vi "STM Read Meta Data (UDP Clst).vi"(6 "Options":T4={"Ignore Timeout Error"=TRUE, "timeout ms (1000)"=1000, "max size (548)"=548}, 8 "error in":errorcluster, 11 "Connection Info In":T2) -> (0 "error out":errorcluster, 1 "Meta data":T1[](array[typedef]), 3 "Connection Info Out":T2, 4 "data info":T3)   [LabVIEW 2014, in "QwaveSys Raspberry Pi Library.lvlib"]
doc: "This VI reads the meta data information from a remote computer. Use this VI to retrieve the variable names and types that a remote computer exports.\n\nThis VI parses the data and returns a cluster containing the meta data information."
uses:
  QwaveSys Raspberry Pi Library.lvlib
  stm_UDP Read Options.ctl
  stm_UDP Data Info.ctl
  stm_UDP Connection Info.ctl
  _SubVIs/stm_MetaDataElement.ctl
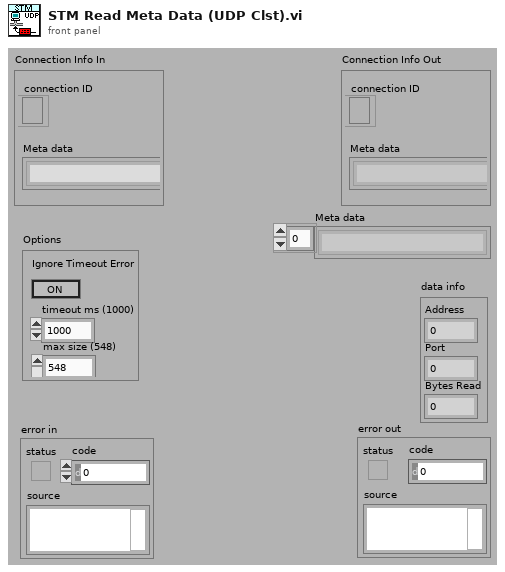
[diagram p1: front panel]
types:
  T1 = typedef "QwaveSys Raspberry Pi Library.lvlib/stm_MetaDataElement.ctl" = string
  T2 = typedef "QwaveSys Raspberry Pi Library.lvlib/stm_UDP Connection Info.ctl" = cluster{"connection ID":refnum<k16>, "Meta data":T1[]}
  T3 = typedef "QwaveSys Raspberry Pi Library.lvlib/stm_UDP Data Info.ctl" = cluster{"Address":u32, "Port":u16, "Bytes Read":i32}
  T4 = typedef "QwaveSys Raspberry Pi Library.lvlib/stm_UDP Read Options.ctl" = cluster{"Ignore Timeout Error":bool, "timeout ms (1000)":i32, "max size (548)":i32}
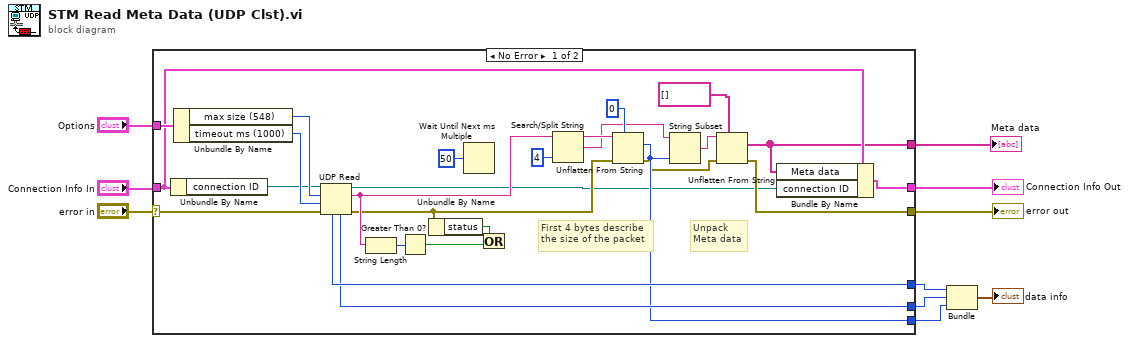
[diagram p0: block diagram]
diagram:
  n1 = case shown="No Error" "error in" {
    selector: "error in" -> [w35 w37]
    tunnel: [w12 _] -> w1
    tunnel: [w36 w37] -> w10
    tunnel: "Connection Info In" -> [w15 w38]
    tunnel: [w16 w38] -> w2
    tunnel: [w28 _] -> w8
    tunnel: [w27 _] -> w7
    tunnel: [w21 _] -> w6
    tunnel: "Options" -> [w17 _]
    frame No Error {
      # "First 4 bytes describe\nthe size of the packet"
      # "Unpack\nMeta data"
      n2 = Unbundle By Name(w15) -> ("connection ID"=w18:refnum<k16>)
      n3 = Unbundle By Name(w17) -> ("max size (548)"=w20:i32, "timeout ms (1000)"=w19:i32)
      n4 = UDP Read(connection ID=w18, max size (548)=w20, timeout ms (25000)=w19, 8:w35) -> (data out=w34:string, error out=w22:errorcluster, 3:w14:refnum<k16>, 4:w27:u16, 6:w28:u32)
      n5 = String Length(string=w34) -> (length=w25:i32)
      n6 = Greater Than 0?(x=w25) -> (x > 0?=w24:bool)
      n7 = Unbundle By Name(w22) -> ("status"=w26:bool)
      n8 = Wait Until Next ms Multiple(millisecond multiple=u32 50) -> ()  [unwired: 1 out]
      n9 = Or(x=w26, y=w24) -> ()  [unwired: 1 out]
      n10 = Search/Split String(string=w34, offset (0)=4) -> (substring before match=w32:string, match + rest of string=w29:string)  [unwired: 2 out]
      n11 = Unflatten From String(type=0, binary string=w32, error in (no error)=w22) -> (value=w21:i32, error out=w11:errorcluster)  [unwired: 3 out]
      n12 = String Subset(string=w29, length (rest)=w21) -> (substring=w30:string)  [unwired: 1 out]
      n13 = Unflatten From String(type=T1[] [] ("Meta data"), binary string=w30, error in (no error)=w11) -> (value=w12:T1[], error out=w36:errorcluster)  [unwired: 3 out]
      n14 = Bundle By Name(cluster=w15, "Meta data"=w12, "connection ID"=w14) -> (w16:T2)
    }
    frame Error {
    }
  }
  "error out" <- w10
  "Connection Info Out" <- w2
  "Meta data" <- w1
  n15 = Bundle("address"=w8, "port"=w7, w6) -> (→"data info":cluster{"address":u32, "port":u16, i32})  [unwired: 1 out]
